vi "part7.vi"() -> ()   [LabVIEW 2009]
panel:
  in  "Array":bool[](array[boolean])
  in  "stop":bool
  # "Outputting to a DC SSR to control a DC load"
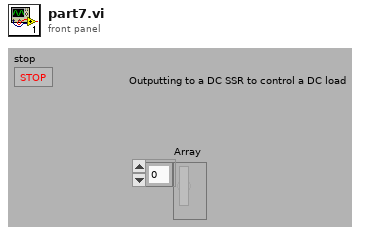
[diagram p1: front panel]
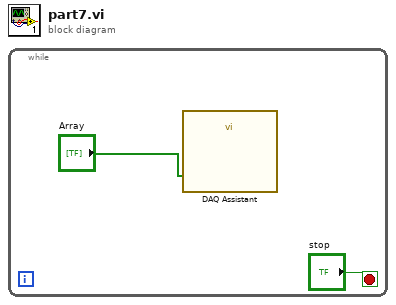
[diagram p0: block diagram]
diagram:
  n1 = while {
    stop <- "stop" stop-if-true
    n2 = call "DAQ Assistant"("data"="Array") -> ()  [unwired: 17 in, 2 out]
  }
